vi "Create.vi"(6 "LabPack Shared Library":path=path "", 8 "Error In":errorcluster) -> (0 "Error Out":errorcluster, 3 "Writer":refnum<class "Writer.lvclass">)   [LabVIEW 2018, in "Toolkit.lvlib" / "Writer.lvclass"]
doc: "Creates a default object of the Writer class for writing and encoding MessagePack data."
uses:
  Writer.lvclass
  Writer.lvclass/Writer.ctl
  Status/Read Is Error.vi
  Status/Read Status.vi
  Status/Read Status Message.vi
  Utility/Status Code.vi
  <vilib>/Utility/error.llb/Error Cluster From Error Code.vi
  Toolkit.lvlib
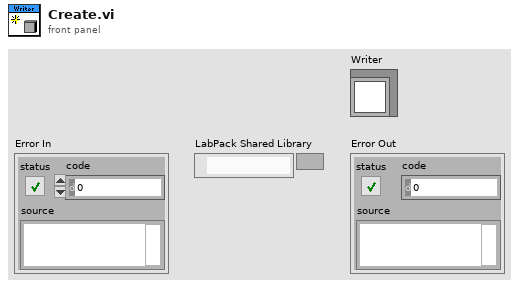
[diagram p1: front panel]
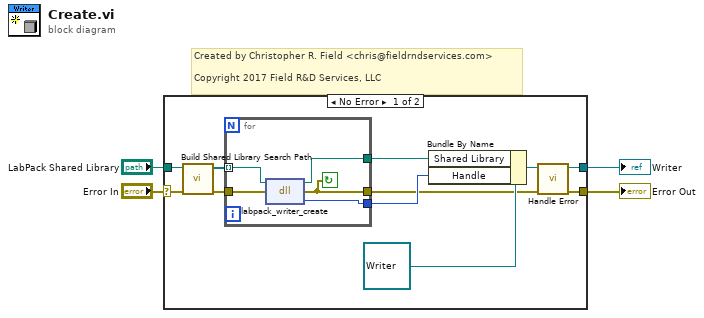
[diagram p0: block diagram]
diagram:
  # "Created by Christopher R. Field <chris@fieldrndservices.com>\n\nCopyright 2017 Field R&D Services, LLC"
  n1 = case shown="No Error" "Error In" {
    selector: "Error In" -> [w10 w21]
    tunnel: [w5 w21] -> w3
    tunnel: [w7 _] -> w2
    tunnel: "LabPack Shared Library" -> [w11 _]
    frame No Error {
      n2 = call "Build Shared Library Search Path.vi"("Error In"=w10, "LabPack Shared Library"=w11) -> ("Error Out"=w9:errorcluster, "Search Path"=w8:path[])  [unwired: 8 in]
      n3 = for {
        tunnel: [w20] -> w13
        tunnel: [w19] -> w12
        tunnel: w8 -> [w17] mode=indexing
        tunnel: w9 -> [w18]
        tunnel: [w16] -> w6
        stop <- w16 continue-if-true
        n4 = dll-call lib="D:/Users/cfield/Code/MessagePack/LabPack/LabVIEW/trunk/src/LabPack/Private/labpack-x64.dll" fn="labpack_writer_create"(path in=w17, error in=w18) -> (path out=w20:path, error out=w16:errorcluster, "return type"=w19:u64)  [unwired: 1 in]
      }
      n5 = Bundle By Name(cluster=refnum<class "Writer.lvclass"> refnum ("LabPack.lvlib:Writer.lvclass"), "Shared Library"=w13, "Handle"=w12) -> (w14:refnum<class "Writer.lvclass">)
      n6 = call "Handle Error.vi"("Error In"=w6, "Writer In"=w14) -> ("Error Out"=w5:errorcluster, "Writer Out"=w7:refnum<class "Writer.lvclass">)  [unwired: 8 in]
    }
    frame Error {
    }
  }
  "Error Out" <- w3
  "Writer" <- w2
